vi "ODMR sweep new.vi"() -> ()   [LabVIEW 2011]
uses:
  <vilib>/DAQmx/read.llb/DAQmx Read (Counter 1D DBL 1Chan NSamp).vi
  <vilib>/DAQmx/write.llb/DAQmx Write (Digital Bool 1Line 1Point).vi
  <vilib>/DAQmx/create/channels.llb/DAQmx Create Channel (DO-Digital Output).vi
  <vilib>/DAQmx/create/channels.llb/DAQmx Create Channel (CI-Count Edges).vi
  <vilib>/DAQmx/configure/timing.llb/DAQmx Timing (Sample Clock).vi
  <vilib>/Utility/file.llb/Write To Spreadsheet File (DBL).vi
  <vilib>/DAQmx/miscellaneous.llb/DAQmx Fill In Error Info.vi
  Program Files/National Instruments/LabVIEW 2011/resource/objmgr/daqmx.rc
panel:
  out "XY Graph":cluster{"Y":dbl[], "Y":dbl[]}[](graph)
  out "Frequency":dbl
  in  "band (1-26.5:2) 2":i32(ring)=2
  in  "resolution (10 Hz:2) 2":i32(ring)=2 items=["0.1 Hz", "1 Hz", "10 Hz", "100 Hz", "1 KHz", "10 KHz", "100 KHz", "1 MHz", "10 MHz", "100 MHz", "1 GHz"]
  in  "GPIB address 2":string="19"
  in  "Freq max":ext=3300000000.0
  in  "Tracking interval":dbl=150.0
  in  "file path (dialog if empty)":path=path "C:/Users/Ouyang Group/Documents/Calibration pictures/Nanodiamond/1-8-14/X=66 Y=92 Pulse ODMR sweep 4"
  out "Z Position":dbl=31.0
  out "Y Position":dbl=62.0
  out "X Position":dbl=97.0
  in  "Z Pos":dbl=31.0
  in  "Y Pos":dbl=97.0
  in  "X Pos":dbl=62.0
  in  "Y Parameters":T1={"Number of Y Steps"=200, "Max Y (V)"=1.0, "Min Y (V)"=-1.0}
  in  "X Parameters":T2={"Number of X Steps"=200, "Max X (V)"=1.0, "Min X (V)"=-1.0}
  in  "RS232 settings":cluster{"Portnumber":i32, "Baudrate":u16}={"Portnumber"=12, "Baudrate"=5} {"Portnumber" items=["COM1", "COM2", "COM3", "COM4", "COM5", "COM6", "COM7", "COM8", "COM9", "COM10", "COM11", "COM12", "COM13", "COM14", "COM15", "COM16", "COM17", "COM18", "COM19", "COM20", "COM21", "COM22", "COM23", "COM24", "COM25", "COM26", "COM27", "COM28", "COM29", "COM30"]; "Baudrate" items=["9600", "14400", "19200", "38400", "57600", "115200"]}
  in  "samples per channel":i32=500
  in  "rate":dbl=100.0 format="%0.2f"
  out "stop":bool
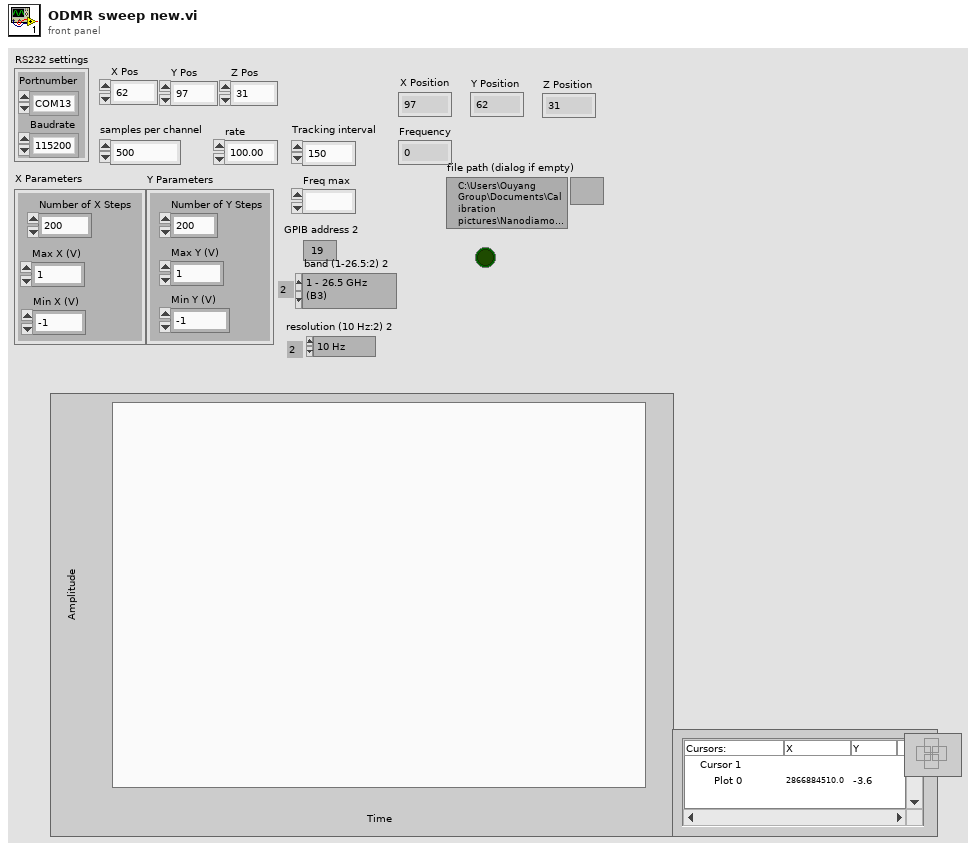
[diagram p1: front panel]
types:
  T1 = cluster{"Number of Y Steps":i32, "Max Y (V)":dbl, "Min Y (V)":dbl}
  T2 = cluster{"Number of X Steps":i32, "Max X (V)":dbl, "Min X (V)":dbl}
  T3 = cluster{"source lock":bool, "lock frequency (Hz)":ext, "coarse tune":bool}
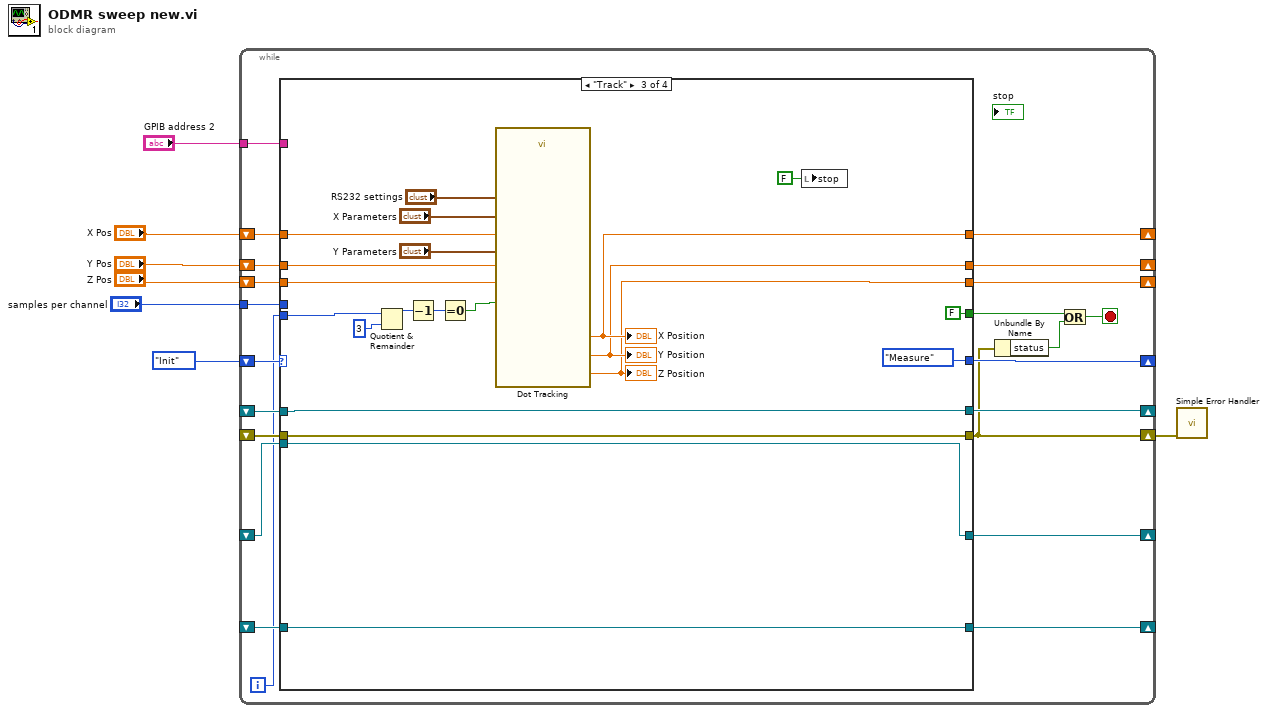
[diagram p0: block diagram]
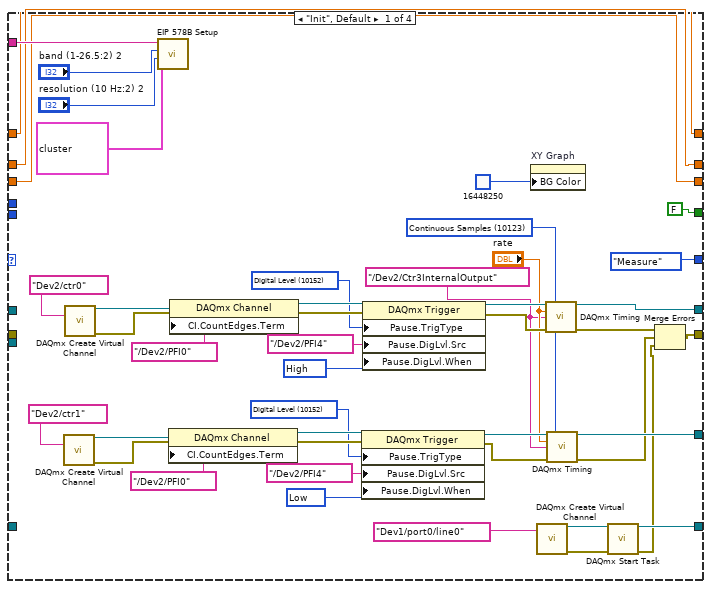
[diagram p2: hidden frame]
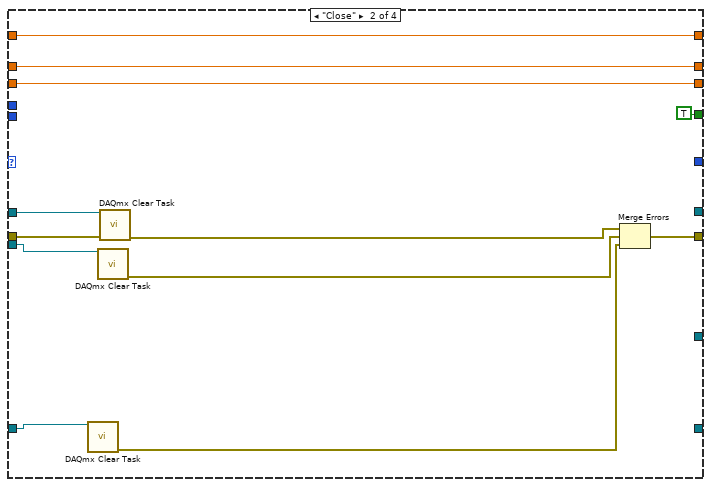
[diagram p3: hidden frame]
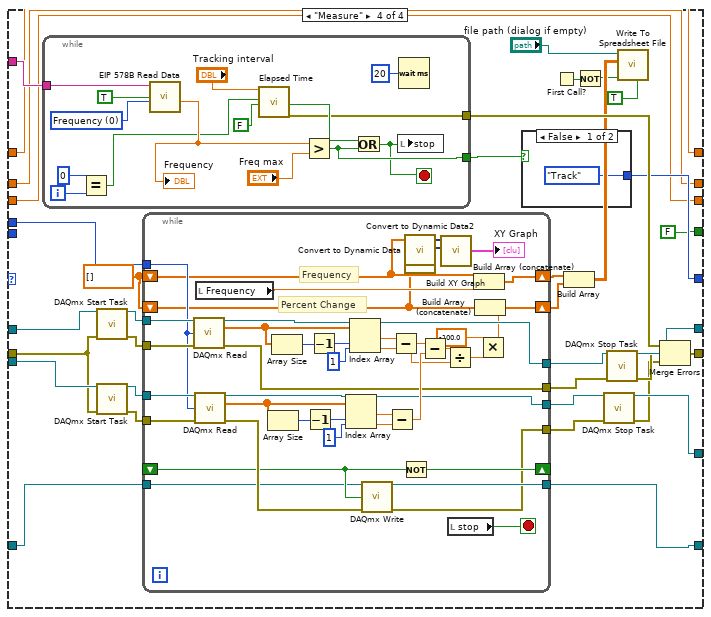
[diagram p4: hidden frame]
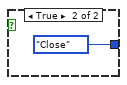
[diagram p5: hidden frame]
diagram:
  n1 = while {
    shift-right: [w25] -> _
    shift-left: enum16{"Init", "Measure", "Track", "Close"}."Init" -> [w29]
    tunnel: "GPIB address 2" -> [w28]
    shift-right: [w27] -> _
    shift-left: _ -> [w24]
    shift-right: [w26] -> _
    shift-left: _ -> [w23]
    shift-right: [w18] -> w4
    shift-left: _ -> [w22]
    shift-right: [w21] -> _
    shift-left: _ -> [w20]
    tunnel: "samples per channel" -> [w15]
    shift-right: [w10] -> _
    shift-left: "X Pos" -> [w13]
    shift-right: [w9] -> _
    shift-left: "Y Pos" -> [w12]
    shift-right: [w8] -> _
    shift-left: "Z Pos" -> [w11]
    i -> [w19]
    stop <- w17 stop-if-true
    n2 = case shown="\"Track\"" w29 {
      tunnel: [FALSE TRUE FALSE FALSE] -> w16
      tunnel: w28 -> [w71 _ _ w142]
      tunnel: [w45 _ w107 w125] -> w27
      tunnel: [w44 _ w106 w122] -> w26
      tunnel: [w41 w79 w96 w141] -> w18
      tunnel: [enum16{"Init", "Measure", "Track", "Close"}."Measure" _ enum16{"Init", "Measure", "Track", "Close"}."Measure" w138] -> w25
      tunnel: w24 -> [_ w85 w107 w134]
      tunnel: w23 -> [_ w83 w106 w131]
      tunnel: w22 -> [_ w84 w96 w129]
      tunnel: [w35 _ w105 w126] -> w21
      tunnel: w20 -> [_ w82 w105 w127]
      tunnel: w19 -> [_ _ w97 _]
      tunnel: w15 -> [_ _ _ w112]
      tunnel: w13 -> [w32 w77 w92 w110]
      tunnel: w12 -> [w31 w76 w91 w109]
      tunnel: w11 -> [w30 w75 w90 w108]
      tunnel: [w32 w77 w89 w110] -> w10
      tunnel: [w31 w76 w88 w109] -> w9
      tunnel: [w30 w75 w87 w108] -> w8
      frame "Init", Default {
        w46 = tag "/Dev2/Ctr3InternalOutput" ("source")
        w48 = 10123 items=["Finite Samples"=10178, "Continuous Samples"=10123, "Hardware Timed Single Point"=12522] ("sample mode")
        w53 = 10214 items=["High"=10192, "Low"=10214] ("Pause.DigLvl.When")
        w55 = 10152 items=["Analog Level"=10101, "Analog Window"=10103, "Digital Level"=10152, "Digital Pattern"=10398, "None"=10230] ("Pause.TrigType")
        w62 = 10192 items=["High"=10192, "Low"=10214] ("Pause.DigLvl.When")
        w64 = 10152 items=["Analog Level"=10101, "Analog Window"=10103, "Digital Level"=10152, "Digital Pattern"=10398, "None"=10230] ("Pause.TrigType")
        n3 = call-poly <vilib>:"DAQmx Create Virtual Channel.vi"("counter"=tag "Dev2/ctr1") -> ("task out"=w60:refnum<k21>, "error out"=w59:errorcluster)  [unwired: 13 in]
        n4 = call-poly <vilib>:"DAQmx Create Virtual Channel.vi"("counter"=tag "Dev2/ctr0") -> ("task out"=w69:refnum<k21>, "error out"=w68:errorcluster)  [unwired: 13 in]
        n5 = call <instrlib>:"EIP 578B Setup.vi"("GPIB Address"=w71, "band (1-26.5 GHz:20)"="band (1-26.5:2) 2", "resolution (1 Hz:1)"="resolution (10 Hz:2) 2", "source locking"=T3 {"source lock"=FALSE, "lock frequency (Hz)"=1000000000.0, "coarse tune"=TRUE}) -> ()  [unwired: 2 in, 2 out]
        n6 = property class="DAQmx Channel"(reference=w60, error in=w59, "CI.CountEdges.Term"=tag "/Dev2/PFI0") -> (reference out=w57:refnum<k21>, error out=w56:errorcluster)
        n7 = property class="DAQmx Channel"(reference=w69, error in=w68, "CI.CountEdges.Term"=tag "/Dev2/PFI0") -> (reference out=w66:refnum<k21>, error out=w65:errorcluster)
        n8 = property class="DAQmx Trigger"(reference=w57, error in=w56, "Pause.TrigType"=w55, "Pause.DigLvl.Src"=tag "/Dev2/PFI4", "Pause.DigLvl.When"=w53) -> (reference out=w50:refnum<k21>, error out=w49:errorcluster)
        n9 = property class="DAQmx Trigger"(reference=w66, error in=w65, "Pause.TrigType"=w64, "Pause.DigLvl.Src"=tag "/Dev2/PFI4", "Pause.DigLvl.When"=w62) -> (reference out=w52:refnum<k21>, error out=w51:errorcluster)
        n10 = property on="XY Graph" class="XYGraph (strict)"("BG Color"=u32 16448250) -> ()  [unwired: 2 in, 2 out]
        n11 = call-poly <vilib>:"DAQmx Create Virtual Channel.vi"("lines"=tag "Dev1/port0/line0") -> ("task out"=w37:refnum<k21>, "error out"=w36:errorcluster)  [unwired: 13 in]
        n12 = call-poly <vilib>:"DAQmx Timing.vi"("task/channels in"=w52, "sample mode"=w48, "rate"="rate", "source"=w46, "error in"=w51) -> ("task out"=w45:refnum<k21>, "error out"=w43:errorcluster)  [unwired: 9 in]
        n13 = call-poly <vilib>:"DAQmx Timing.vi"("task/channels in"=w50, "sample mode"=w48, "rate"="rate", "source"=w46, "error in"=w49) -> ("task out"=w44:refnum<k21>, "error out"=w42:errorcluster)  [unwired: 9 in]
        n14 = call <vilib>:"DAQmx Start Task.vi"("task/channels in"=w37, "error in"=w36) -> ("task out"=w35:refnum<k21>, "error out"=w34:errorcluster)  [unwired: 12 in]
        n15 = Merge Errors(w43, w42, w34) -> (w41:errorcluster)
      }
      frame "Close" {
        n16 = call <vilib>:"DAQmx Clear Task.vi"("task in"=w82) -> ("error out"=w80:errorcluster)  [unwired: 14 in]
        n17 = call <vilib>:"DAQmx Clear Task.vi"("task in"=w83) -> ("error out"=w81:errorcluster)  [unwired: 14 in]
        n18 = call <vilib>:"DAQmx Clear Task.vi"("task in"=w85, "error in"=w84) -> ("error out"=w78:errorcluster)  [unwired: 13 in]
        n19 = Merge Errors(w78, w81, w80) -> (w79:errorcluster)
      }
      frame "Track" {
        n20 = Quotient & Remainder(x=w97, y=3) -> (x-y*floor(x/y)=w100:i32)  [unwired: 1 out]
        n21 = Decrement(x=w100) -> (x-1=w101:i32)
        n22 = Equal To 0?(x=w101) -> (x = 0?=w98:bool)
        n23 = call "Dot Tracking.vi"("X Parameters"="X Parameters", "Y Parameters"="Y Parameters", "RS232 settings"="RS232 settings", "X Pos"=w92, "Y pos"=w91, "Z Pos"=w90, "Z-track?"=w98) -> ("X Position"=w89:dbl, "Y Position"=w88:dbl, "Z Position"=w87:dbl)  [unwired: 2 in, 4 out]
        "X Position" <- w89
        "Y Position" <- w88
        "Z Position" <- w87
        n24 = local write "stop"(FALSE ("stop")) -> ()
      }
      frame "Measure" {
        w111 = dbl[] []
        n25 = while {
          tunnel: [w197] -> w139
          tunnel: w142 -> [w194]
          tunnel: [w193] -> w140
          i -> [w189]
          stop <- w186 stop-if-true
          w196 = 0 items=["Frequency", "Power", "Both"] ("output mode (freq:0)")
          n26 = Equal?(x=0, y=w189) -> (x = y?=w187:bool)
          n27 = call <instrlib>:"EIP 578B Read Data.vi"("output mode (freq:0)"=w196, "fast (T=active)"=TRUE, "GPIB"=w194) -> ("frequency (Hz)"=w191:ext)  [unwired: 1 in, 3 out]
          "Frequency" <- w191
          n28 = call "Elapsed Time"("Time Target (s)"="Tracking interval", "Reset"=w187, "Auto Reset"=FALSE) -> ("Time has Elapsed"=w199:bool, "error out"=w193:errorcluster)  [unwired: 9 in, 6 out]
          n29 = Greater?(x=w191, y="Freq max") -> (0:w197:bool)
          n30 = Or(x=w199, y=w197) -> (x .or. y?=w186:bool)
          n31 = local write "stop"(w186) -> ()
          n32 = Wait (ms)(milliseconds to wait=u32 20) -> ()  [unwired: 1 out]
        }
        n33 = call <vilib>:"DAQmx Start Task.vi"("task/channels in"=w134, "error in"=w129) -> ("task out"=w132:refnum<k21>, "error out"=w133:errorcluster)  [unwired: 12 in]
        n34 = call <vilib>:"DAQmx Start Task.vi"("task/channels in"=w131, "error in"=w129) -> ("task out"=w130:refnum<k21>, "error out"=w128:errorcluster)  [unwired: 12 in]
        n35 = while {
          shift-right: [w171] -> w118
          shift-left: w111 -> [w149]
          shift-right: [w170] -> w119
          shift-left: w111 -> [w151]
          shift-right: [w164] -> _
          shift-left: _ -> [w165]
          tunnel: w130 -> [w163]
          tunnel: [w162] -> w124
          tunnel: [w161] -> w136
          tunnel: [w155] -> w135
          tunnel: w133 -> [w160]
          tunnel: w132 -> [w159]
          tunnel: w128 -> [w158]
          tunnel: w127 -> [w157]
          tunnel: [w156] -> w126
          tunnel: [w154] -> w121
          tunnel: w112 -> [w153]
          stop <- w185 stop-if-true
          # "Percent Change"
          # "Frequency"
          n36 = call-poly <vilib>:"DAQmx Read.vi"("task/channels in"=w159, "number of samples per channel"=w153, "error in"=w160) -> ("task out"=w161:refnum<k21>, "data"=w184:dbl[], "error out"=w162:errorcluster)  [unwired: 10 in]
          n37 = call-poly <vilib>:"DAQmx Read.vi"("task/channels in"=w163, "number of samples per channel"=w153, "error in"=w158) -> ("task out"=w155:refnum<k21>, "data"=w173:dbl[], "error out"=w166:errorcluster)  [unwired: 10 in]
          n38 = local read "Frequency"() -> (w152:dbl)
          n39 = Array Size(array=w173) -> (size(s)=w178:i32)
          n40 = Array Size(array=w184) -> (size(s)=w183:i32)
          n41 = Decrement(x=w178) -> (x-1=w177:i32)
          n42 = Decrement(x=w183) -> (x-1=w182:i32)
          n43 = Index Array(array=w173, index #1=w177, index #2=1 ("index")) -> (element #1=w174:dbl, element #2=w175:dbl)
          n44 = Index Array(array=w184, index #1=w182, index #2=1 ("index")) -> (element #1=w179:dbl, element #2=w180:dbl)
          n45 = call-poly <vilib>:"DAQmx Write.vi"("task/channels in"=w157, "data"=w165, "error in"=w166) -> ("task out"=w156:refnum<k21>, "error out"=w154:errorcluster)  [unwired: 10 in, 1 out]
          n46 = Subtract(x=w174, y=w175) -> (x-y=w172:dbl)
          n47 = Subtract(x=w179, y=w180) -> (x-y=w168:dbl)
          n48 = Not(x=w165) -> (.not. x?=w164:bool)
          n49 = call "Convert to Dynamic Data"("Array"=w151) -> ("Dynamic Data Type"=w150:dynamicdata)  [unwired: 3 in]
          n50 = call "Convert to Dynamic Data2"("Array"=w149) -> ("Dynamic Data Type"=w148:dynamicdata)  [unwired: 3 in]
          n51 = Subtract(x=w168, y=w172) -> (x-y=w169:dbl)
          n52 = call "Build XY Graph"("Y Input"=w148, "X Input"=w150) -> ("XY Graph"=→"XY Graph":cluster{"Y":dbl[], "Y":dbl[]}[])  [unwired: 3 in, 6 out]
          n53 = Divide(x=w169, y=w168) -> (x/y=w167:dbl)
          n54 = local read "stop"() -> (w185:bool)
          n55 = Build Array (concatenate)(w151, w152) -> (w170:dbl[])
          n56 = Multiply(x=-100.0, y=w167) -> (x*y=w146:dbl)
          n57 = Build Array (concatenate)(w149, w146) -> (w171:dbl[])
        }
        n58 = case shown="False" w139 {
          tunnel: [enum16{"Init", "Measure", "Track", "Close"}."Track" enum16{"Init", "Measure", "Track", "Close"}."Close"] -> w138
          frame False {
          }
          frame True {
          }
        }
        n59 = First Call?() -> (First Call?: T/F=w116:bool)
        n60 = Build Array(w119, w118) -> (w117:dbl[][])
        n61 = Not(x=w116) -> (.not. x?=w115:bool)
        n62 = call <vilib>:"DAQmx Stop Task.vi"("task/channels in"=w135, "error in"=w121) -> ("task out"=w122:refnum<k21>, "error out"=w120:errorcluster)  [unwired: 12 in]
        n63 = call <vilib>:"DAQmx Stop Task.vi"("task/channels in"=w136, "error in"=w124) -> ("task out"=w125:refnum<k21>, "error out"=w123:errorcluster)  [unwired: 12 in]
        n64 = call-poly <vilib>:"Write To Spreadsheet File.vi"("transpose? (no:F)"=TRUE, "append to file? (new file:F)"=w115, "2D data"=w117, "file path (dialog if empty)"="file path (dialog if empty)") -> ()  [unwired: 4 in, 1 out]
        n65 = Merge Errors(w140, w123, w120) -> (w141:errorcluster)
      }
    }
    n66 = Unbundle By Name(w18) -> ("status"=w14:bool)
    n67 = Or(x=w16, y=w14) -> (x .or. y?=w17:bool)
  }
  n68 = call <vilib>:"Simple Error Handler.vi"("error in (no error)"=w4) -> ()  [unwired: 4 in, 5 out]
